vi "Contants.vi"() -> ()   [LabVIEW 2019]
panel:
  in  "Closed Ramp DRIVE":dbl
  in  "Open Ramp DRIVE":dbl
  in  "PIDVal DRIVE":T1
  in  "MotionMagic Config DRIVE":T2
  in  "Closed Ramp":dbl
  in  "Open Ramp":dbl
  in  "PIDVal":T1
  in  "MotionMagic Config":T2
  # "Shooter"
  # "DRIVE"
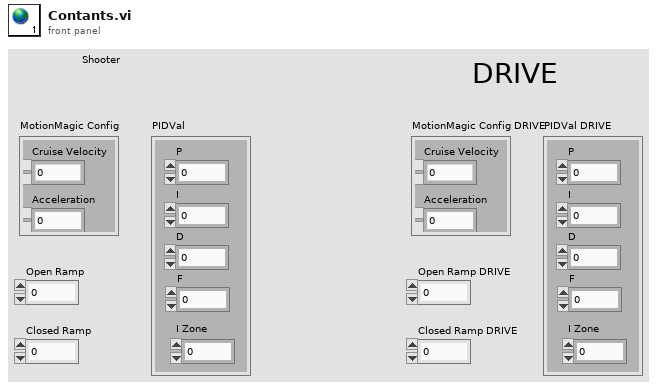
[diagram p1: front panel]
types:
  T1 = cluster{"P":dbl, "I":dbl, "D":dbl, "F":dbl, "I Zone":dbl}
  T2 = cluster{"Cruise Velocity":i32, "Acceleration":i32}
diagram:
